vi "free_c_string_at_memory_address.vi"(8 "error in (no error)":errorcluster, 11 "memory_address":u64) -> (0 "error out":errorcluster)   [LabVIEW 2020, in "reqwest.lvlib"]
uses:
  reqwest.lvlib
  lv_reqwest_64.so
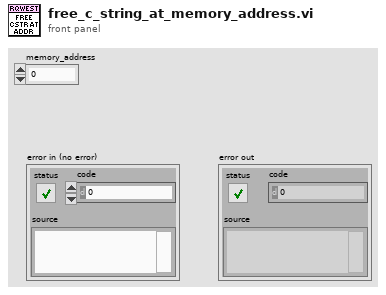
[diagram p1: front panel]
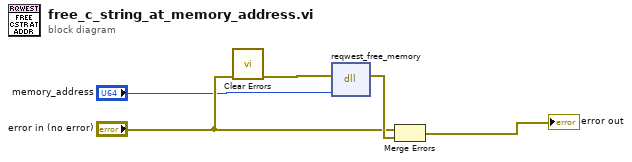
[diagram p0: block diagram]
diagram:
  n1 = call <vilib>:"Clear Errors.vi"("error in (no error)"="error in (no error)") -> ("error out"=w2:errorcluster)  [unwired: 5 in, 1 out]
  n2 = dll-call lib="home/jim-kring/Projects/reqwest-rs-labview/lv_src/lv_reqwest_64.so" fn="reqwest_free_memory"(error in=w2, "ptr"="memory_address") -> (error out=w4:errorcluster)  [unwired: 4 in, 1 out]
  n3 = Merge Errors("error in (no error)", w4) -> (→"error out":errorcluster)
